vi "General measurements.vi"(4 "Limit":dbl=0.01, 5 "Number of averages":u32=10) -> ()   [LabVIEW 2018]
doc: "This example demonstrates how to retreive Real 64 data from the instrument and how to use the Real 64 Converter VI to convert this data into an array of doubles.\n\nThis example demonstrates the following:\n• Clearing and configuring a non-volatile reading buffer\n• Quickly seting up the source\n• Quickly configuring the measure hardware\n• Take measurements into a reading buffer\n• Configure the data output format\n• Print back a reading buffer\n• Convert the returned data into an array of doubles"
uses:
  Program Files/National Instruments/LabVIEW 2023/instr.lib/Keithley 2600 Series old/Keithley 2600 Series.lvlib
  <vilib>/Utility/file.llb/Write Delimited Spreadsheet (DBL).vi
  <vilib>/Utility/file.llb/Read Delimited Spreadsheet (DBL).vi
  <vilib>/Analysis/NI_AALBase.lvlib
  <vilib>/Analysis/6fits.llb/Curve Fitting Criteria.ctl
  <vilib>/Analysis/NI_AALPro.lvlib
  Program Files/National Instruments/LabVIEW 2023/instr.lib/Keithley 2600 Series old/Public/Channel.ctl
panel:
  out "slope^-1":dbl
  out "residual":dbl
  out "intercept":dbl
  out "slope":dbl
  in  "Multiplier":dbl=1.0
  out "y/x":dbl
  out "x/y":dbl
  in  "Load":bool
  in  "Save":bool
  in  "Append":bool
  in  "Fill":bool
  in  "Filename":path
  in  "Save":bool
  in  "Steps":i32=50
  in  "To":dbl=0.1 format="%#_13g"
  in  "From":dbl=-0.1 format="%#_13g"
  in  "Channel":T1
  out "XY Graph":T2(graph)
  in  "Values":dbl[](array[numeric])=[-0.1, -0.096, -0.092, -0.08800000000000001, -0.084, -0.08, -0.07600000000000001, -0.07200000000000001, -0.068, -0.064, -0.060000000000000005, -0.05600000000000001, -0.052000000000000005, -0.048, -0.044000000000000004, -0.04000000000000001, -0.036000000000000004, -0.032, -0.027999999999999997, -0.024000000000000007, -0.020000000000000004, -0.016, -0.01200000000000001, -0.008000000000000007, -0.0040000000000000036, 0.0, 0.0040000000000000036, 0.007999999999999993, 0.011999999999999997, 0.016, 0.01999999999999999, 0.023999999999999994, 0.027999999999999997, 0.032, 0.036000000000000004, 0.04000000000000001, 0.04400000000000001, 0.04799999999999999, 0.05199999999999999, 0.055999999999999994, 0.06, 0.064, 0.068, 0.07200000000000001, 0.07599999999999998, 0.07999999999999999, 0.08399999999999999, 0.088, 0.092, 0.096, 0.1]
  in  "Sense (2 Wire)":enum32{"2 Wire", "4 Wire", "Calibration"}(ring)
  out "SD":dbl=4.353305074225212e-09 format="%e"
  out "mean":dbl=1.7599910506760354e-08 format="%e"
  in  "Source":enum32{"Current", "Voltage"}(ring)=enum."Voltage"
  in  "Measure":T3(ring)
  in  "Start":bool
  in  "stop":bool
  out "Driving signal":dbl[](graph)
  # "Instrument setup"
  # "Input values"
  # "Linear Fit"
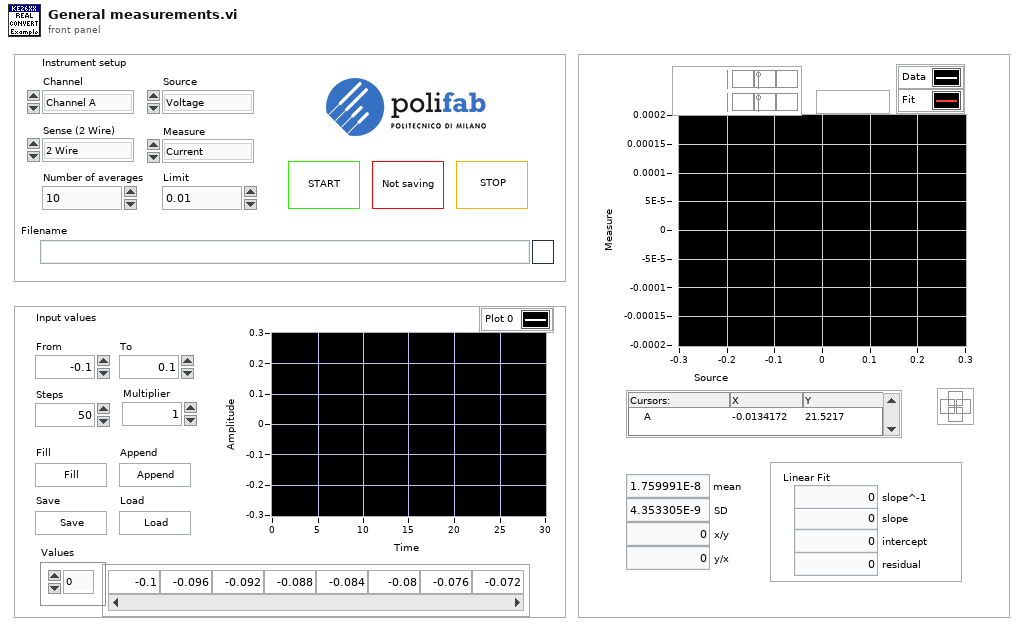
[diagram p1: front panel]
types:
  T1 = typedef "Keithley 2600 Series.lvlib/Channel.ctl" = enum32{"Channel A", "Channel B"}
  T2 = cluster{"Data Array Out":dbl[], "Data Array Out":dbl[]}[]
  T3 = enum32{"Current", "Voltage", "IV", "Resistance", "Power"}
  T4 = typedef "NI_AALPro.lvlib/Curve Fitting Criteria.ctl" = u16
  T5 = cluster{"Data Array Out":dbl[], "Data Array Out":dbl[]}
  T6 = cluster{"Data Array Out":dbl[], "Best Linear Fit":dbl[]}
  T7 = cluster{"Data Array Out":dbl[], "Best Linear Fit":dbl[]}[]
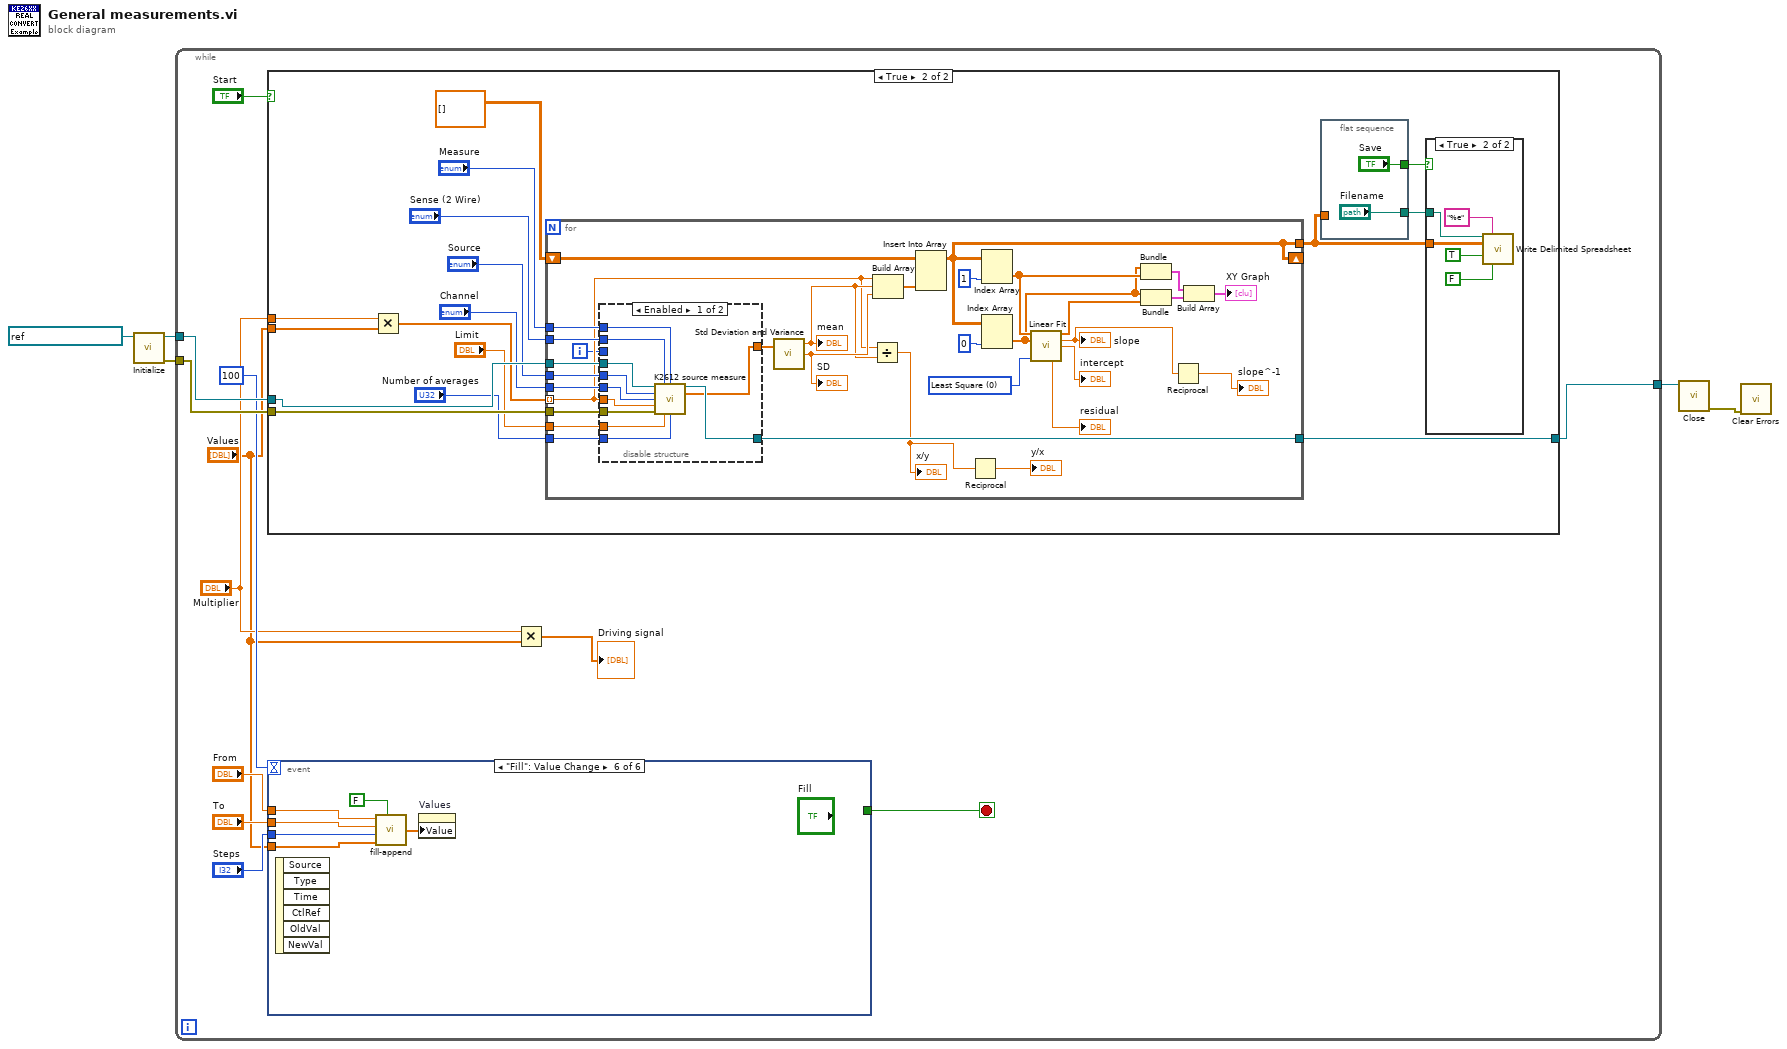
[diagram p0: block diagram]
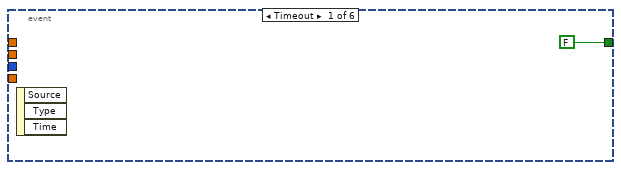
[diagram p2: hidden frame]
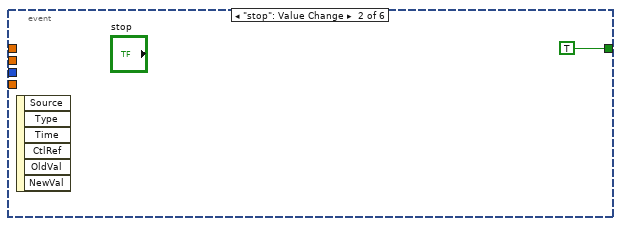
[diagram p3: hidden frame]
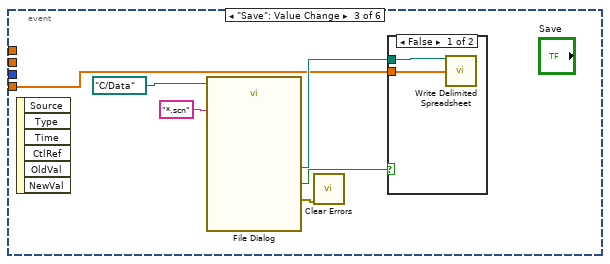
[diagram p4: hidden frame]
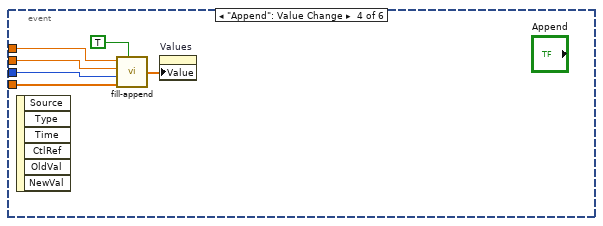
[diagram p6: hidden frame]
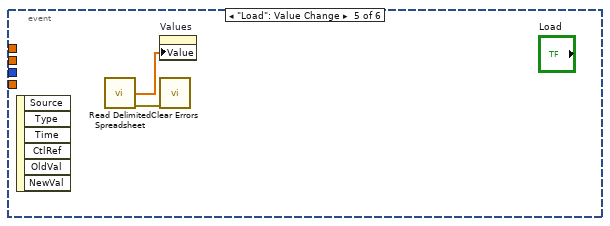
[diagram p7: hidden frame]
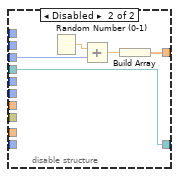
[diagram p10: hidden frame]
diagram:
  n1 = call "Initialize.vi"("VISA resource name"=refnum<visa-resource-name> "GPIB0::26::INSTR") -> ("error out"=w4:errorcluster, "VISA resource name out"=w5:refnum<visa-resource-name>)  [unwired: 5 in, 4 out]
  n2 = while {
    tunnel: w5 -> [w17]
    tunnel: w4 -> [w16]
    tunnel: [w15] -> w2
    stop <- w10 stop-if-true
    n3 = case shown="True" "Start" {
      tunnel: w17 -> [w42 w58]
      tunnel: w16 -> [_ w57]
      tunnel: [w42 w53] -> w15
      tunnel: "Values" -> [_ w45]
      tunnel: "Multiplier" -> [_ w43]
      frame False {
      }
      frame True {
        n4 = Multiply(x=w43, y=w45) -> (x*y=w44:dbl[])
        n5 = for {
          tunnel: w57 -> [w96]
          tunnel: "Source" -> [w95]
          tunnel: "Number of averages" -> [w94]
          tunnel: w44 -> [w80] mode=indexing
          tunnel: "Limit" -> [w93]
          tunnel: "Measure" -> [w91]
          tunnel: "Sense (2 Wire)" -> [w89]
          tunnel: w58 -> [w97]
          tunnel: [w92] -> w53
          shift-right: [w77] -> _
          shift-left: dbl[][] [] ("Data Array Out") -> [w88]
          tunnel: "Channel" -> [w87]
          tunnel: [w77] -> w46
          i -> [w68]
          w78 = T4 0 items=["Least Square", "Least Absolute Residual", "Bisquare"] ("method")
          n6 = disable-structure shown="Enabled" {
            disable-tunnel: w97 -> [w108 w113]
            disable-tunnel: w96 -> [w107 _]
            disable-tunnel: w95 -> [w106 _]
            disable-tunnel: w94 -> [w105 _]
            disable-tunnel: w93 -> [w104 _]
            disable-tunnel: [w103 w113] -> w92
            disable-tunnel: w91 -> [w102 _]
            disable-tunnel: [w101 w112] -> w90
            disable-tunnel: w89 -> [w100 _]
            disable-tunnel: w87 -> [w99 _]
            disable-tunnel: w80 -> [w98 _]
            disable-tunnel: w68 -> [_ w111]
            frame Enabled {
              n7 = call "K2612 source measure.vi"("VISA Refnum in"=w108, "Sense (2 Wire)"=w100, "Measure"=w102, "Source"=w106, "Channel"=w99, "Level (5 V)"=w98, "error in (no error)"=w107, "Limit (0.01 A)"=w104, "Measure Count (10)"=w105) -> ("VISA Refnum out"=w103:refnum<visa-resource-name>, "Data Array Out"=w101:dbl[])  [unwired: 5 in]
            }
            frame Disabled {
              n8 = Random Number (0-1)() -> (number: 0 to 1=w110:dbl)
              n9 = Add(x=w110, y=w111) -> (x+y=w109:dbl)
              n10 = Build Array(w109) -> (w112:dbl[])
            }
          }
          n11 = call <vilib>:"Std Deviation and Variance.vi"("X"=w90) -> ("mean"=w83:dbl, "standard deviation"=w86:dbl)  [unwired: 1 in, 1 out]
          "mean" <- w83
          "SD" <- w86
          n12 = Divide(x=w80, y=w83) -> (x/y=w82:dbl)
          "x/y" <- w82
          n13 = Build Array(w80, w83, w86) -> (w85:dbl[])
          n14 = Insert Into Array(array=w88, new element=w85) -> (w77:dbl[][])  [unwired: 2 in]
          n15 = Reciprocal(x=w82) -> (1/x=→"y/x":dbl)
          n16 = Index Array(array=w77, index (col)=1 ("disabled index (col)")) -> (element=w79:dbl[])  [unwired: 1 in]
          n17 = Index Array(array=w77, index (col)=0 ("disabled index (col)")) -> (element=w73:dbl[])  [unwired: 1 in]
          n18 = call <vilib>:"Linear Fit.vi"("Y"=w79, "X"=w73, "method"=w78) -> ("Best Linear Fit"=w72:dbl[], "slope"=w67:dbl, "intercept"=→"intercept":dbl, "residue"=→"residual":dbl)  [unwired: 8 in, 1 out]
          "slope" <- w67
          n19 = Bundle("Data Array Out"=w73, "Data Array Out"=w79) -> (w75:T5)  [unwired: 1 in]
          n20 = Bundle("Data Array Out"=w73, "Best Linear Fit"=w72) -> (w71:T6)  [unwired: 1 in]
          n21 = Reciprocal(x=w67) -> (1/x=→"slope^-1":dbl)
          n22 = Build Array(w75, w71) -> (→"XY Graph":T7)
        }
        n23 = flat-sequence {
          tunnel: ["Save"] -> w48
          tunnel: ["Filename"] -> w47
          tunnel: w46 -> [_]
          frame #0 {
          }
        }
        n24 = case shown="True" w48 {
          tunnel: w47 -> [_ w60]
          tunnel: w46 -> [_ w59]
          frame False {
          }
          frame True {
            n25 = call-poly <vilib>:"Write Delimited Spreadsheet.vi"("file path (dialog if empty)"=w60, "format (%.3f)"="%e", "2D data"=w59, "append to file? (new file:F)"=TRUE, "transpose? (no:F)"=FALSE) -> ()  [unwired: 9 in, 2 out]
          }
        }
      }
    }
    n26 = event shown="[5] \"Fill\": Value Change" {
      selector: _ -> [_ _ _ _ _ _]
      dyn-events: _ -> [_ _ _ _ _ _]
      timeout: u32 100 ("milliseconds to wait") -> [_ _ _ _ _ _]
      tunnel: "Values" -> [_ _ w20 w29 _ w41]
      tunnel: "To" -> [_ _ _ w31 _ w39]
      tunnel: "From" -> [_ _ _ w32 _ w38]
      tunnel: "Steps" -> [_ _ _ w30 _ w37]
      tunnel: [FALSE TRUE _ _ _ _] -> w10
      event Timeout {
        n27 = event-data() -> ()  [unwired: 1 in, 3 out]
      }
      event "stop": Value Change {
        n28 = event-data() -> ()  [unwired: 1 in, 6 out]
      }
      event "Save": Value Change {
        n29 = event-data() -> ()  [unwired: 1 in, 6 out]
        n30 = call "File Dialog"("start path"=path "C:/Data", "pattern (all files)"="*.scn") -> ("selected path"=w23:path, "cancelled"=w22:bool, "error out"=w21:errorcluster)  [unwired: 10 in, 1 out]
        n31 = call <vilib>:"Clear Errors.vi"("error in (no error)"=w21) -> ()  [unwired: 5 in, 2 out]
        n32 = case shown="False" w22 {
          tunnel: w20 -> [w27 _]
          tunnel: w23 -> [w26 _]
          frame False {
            n33 = call-poly <vilib>:"Write Delimited Spreadsheet.vi"("file path (dialog if empty)"=w26, "1D data"=w27) -> ()  [unwired: 12 in, 2 out]
          }
          frame True {
          }
        }
      }
      event "Append": Value Change {
        n34 = event-data() -> ()  [unwired: 1 in, 6 out]
        n35 = call "fill-append.vi"("Append/Fill"=TRUE, "array"=w29, "Steps (max 200)"=w30, "To"=w31, "From"=w32) -> ("appended magnetic field values"=w28:dbl[])  [unwired: 1 in]
        n36 = property on="Values" class="Arr (strict)"("Value"=w28) -> ()  [unwired: 2 in, 2 out]
      }
      event "Load": Value Change {
        n37 = event-data() -> ()  [unwired: 1 in, 6 out]
        n38 = call-poly <vilib>:"Read Delimited Spreadsheet.vi"() -> ("first row"=w34:dbl[], "error out"=w35:errorcluster)  [unwired: 10 in, 4 out]
        n39 = property on="Values" class="Arr (strict)"("Value"=w34) -> ()  [unwired: 2 in, 2 out]
        n40 = call <vilib>:"Clear Errors.vi"("error in (no error)"=w35) -> ()  [unwired: 5 in, 2 out]
      }
      event "Fill": Value Change {
        n41 = event-data() -> ()  [unwired: 1 in, 6 out]
        n42 = call "fill-append.vi"("Append/Fill"=FALSE, "array"=w41, "Steps (max 200)"=w37, "To"=w39, "From"=w38) -> ("appended magnetic field values"=w36:dbl[])  [unwired: 1 in]
        n43 = property on="Values" class="Arr (strict)"("Value"=w36) -> ()  [unwired: 2 in, 2 out]
      }
    }
    n44 = Multiply(x="Multiplier", y="Values") -> (x*y=→"Driving signal":dbl[])
  }
  n45 = call "Close.vi"("VISA resource name"=w2) -> ("error out"=w1:errorcluster)  [unwired: 1 in, 9 out]
  n46 = call <vilib>:"Clear Errors.vi"("error in (no error)"=w1) -> ()  [unwired: 5 in, 2 out]
